vi "Lockin Initialize.vi"(8 "errorIN":errorcluster caption="Error") -> (0 "errorOUT":errorcluster caption="Error", 3 "ready?":bool)   [LabVIEW 2009, in "Lockin SR830.lvclass"]
uses:
  Lockin SR830.lvclass
  Global/GPIB Numbers.vi
panel:
  out "data":string
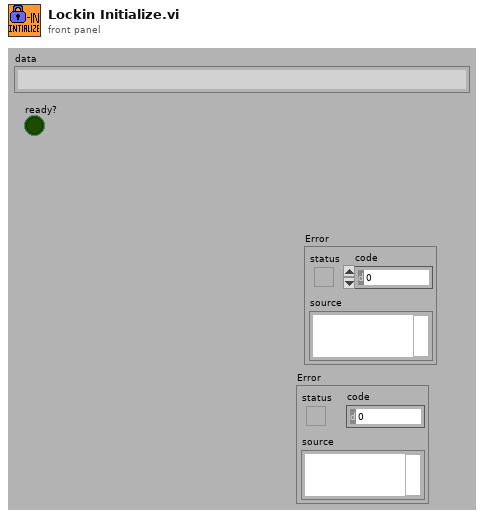
[diagram p1: front panel]
types:
  T1 = typedef "GPIB Type Def.ctl" = cluster{"Name":string, "bus":dbl, "GPIB":dbl, "GPIB as string":string, "byte":i32, "VISA Resource Name":refnum<visa-resource-name>}
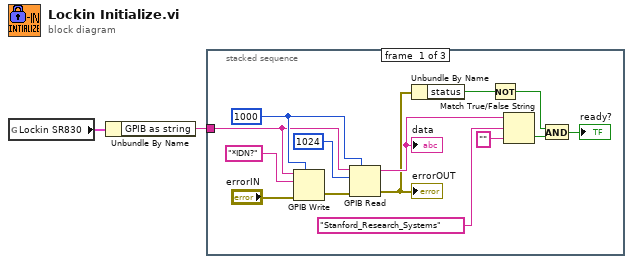
[diagram p0: block diagram]
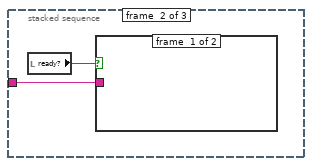
[diagram p2: hidden frame]
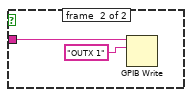
[diagram p3: hidden frame]
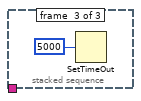
[diagram p4: hidden frame]
diagram:
  n1 = global read "GPIB Numbers.vi" "Lockin SR830"() -> (w1:T1)
  n2 = Unbundle By Name(w1) -> ("GPIB as string"=w2:string)
  n3 = stacked-sequence {
    tunnel: w2 -> [w3 w18 _]
    frame #0 {
      w10 = 1000
      n4 = GPIB Write(0:w3, 1:"*IDN?", 3:"errorIN", 4:w10) -> (6:w15:errorcluster)  [unwired: 2 out]
      n5 = GPIB Read(0:w3, 1:1024, 3:w15, 4:w10) -> (5:w13:string, 7:w4:errorcluster)  [unwired: 2 out]
      "data" <- w13
      "errorOUT" <- w4
      n6 = Unbundle By Name(w4) -> ("status"=w9:bool)
      n7 = Not(x=w9) -> (.not. x?=w6:bool)
      n8 = Match True/False String(2:"", 3:"Stanford_Research_Systems", 4:w13) -> (0:w7:bool)  [unwired: 1 out]
      n9 = And(x=w6, y=w7) -> (x .and. y?=→"ready?":bool)
    }
    frame #1 {
      n10 = local read "ready?"() -> (w17:bool)
      n11 = case shown="True" w17 {
        tunnel: w18 -> [_ w20]
        frame #0 {
        }
        frame #1 {
          n12 = GPIB Write(0:w20, 1:"OUTX 1") -> ()  [unwired: 1 in, 4 out]
        }
      }
    }
    frame #2 {
      n13 = SetTimeOut(1:5000) -> ()  [unwired: 1 out]
    }
  }
